vi "Abort.vi"(7 "Enable Channel 1 to 2":bool, 8 "error in (no error)":errorcluster, 9 "Device Action (0: Acquire)":i32(ring) items=["Acquire", "Transient", "Both"], 10 "Channel List ({Channel1})":i32[](array[ring])=[0] items=["Channel 1", "Channel 2"], 11 "VISA resource name":refnum<visa-resource-name>) -> (0 "error out":errorcluster, 3 "VISA resource name out":refnum<visa-resource-name>)   [LabVIEW 2020, in "Agilent B2900 Series.lvlib"]
doc: "Aborts the specified device action for the specified channel. Trigger status is changed to idle.\n\n<B>Note:</B> Use this VI only with other low-level VIs. The high-level VIs automatically incorporate this functionality. This VI does not check the instrument status."
uses:
  Agilent B2900 Series.lvlib
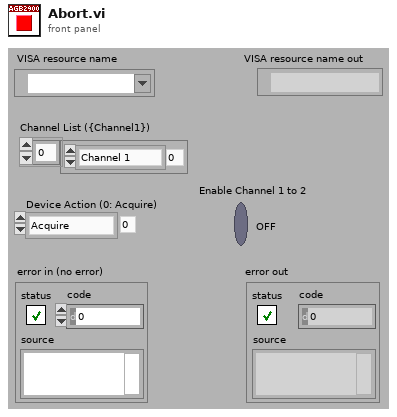
[diagram p1: front panel]
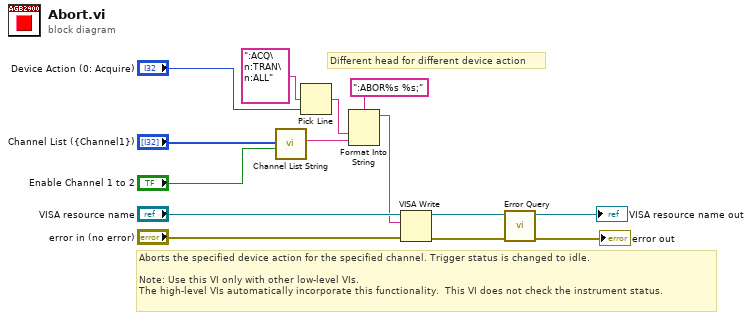
[diagram p0: block diagram]
diagram:
  # "Aborts the specified device action for the specified channel. Trigger status is changed to idle.\n\nNote: Use this VI only with other low-level VIs.  \nThe high-level VIs automatically incorporate this functionality.  This VI does not check the instrument status."
  # "Different head for different device action"
  n1 = call "Channel List String.vi"("Enable Channel 1 to 2"="Enable Channel 1 to 2", "Channel List ({Channel1})"="Channel List ({Channel1})") -> ("Channel List Command String"=w6:string)  [unwired: 9 in]
  n2 = Pick Line(multi-line string=":ACQ\n:TRAN\n:ALL", line index="Device Action (0: Acquire)") -> (output string=w7:string)  [unwired: 1 in]
  n3 = Format Into String(format string=":ABOR%s %s;", w7, w6) -> (resulting string=w10:string)  [unwired: 2 in, 1 out]
  n4 = VISA Write(VISA resource name="VISA resource name", write buffer=w10, error in (no error)="error in (no error)") -> (VISA resource name out=w4:refnum<visa-resource-name>, error out=w2:errorcluster)  [unwired: 1 out]
  n5 = call "Error Query.vi"("error in (no error)"=w2, "VISA resource name"=w4) -> ("error out"=→"error out":errorcluster, "VISA resource name out"=→"VISA resource name out":refnum<visa-resource-name>)  [unwired: 6 in, 2 out]
